vi "CheckCameraAttributes-CDH.vi"(2 "error in":errorcluster, 3 "Camera Name":T1) -> (0 "error out":errorcluster, 1 "Session Out":T1)   [LabVIEW 2013]
doc: "The Grab and Attributes Setup VI acquires images continuously and displays the images in an image control using high-level acquisition VIs. The VI also modifes the camera attributes while acquiring images. A grab is appropriate for high-speed applications in which you need to process only one image at a time."
uses:
  <vilib>/userdefined/High Color/IMAQdx.ctl
  <vilib>/vision/driver/IMAQdx.llb/IMAQdx Attribute Type.ctl
  <vilib>/vision/driver/IMAQdx.llb/IMAQdx Attribute Visibility.ctl
  <vilib>/vision/driver/NI_Vision_Acquisition_Software.lvlib
  <resource>/objmgr/imaqdx.rc
panel:
  out "Trigger::TriggerSource":string
  out "Trigger::TriggerParameter":dbl
  out "TriggerDelay::Value":dbl
  out "Trigger::TriggerActivation":string
  out "Shutter::Value":dbl
  out "Sharpness::Value":dbl
  out "Gamma::Value":dbl
  out "Gain::Value":dbl
  out "FrameRate::Value":dbl
  out "Brightness::Value":dbl
  out "AutoExposure::Value":dbl
  out "TriggerDelay::Mode":string
  out "Trigger::TriggerMode":string
  out "Shutter::Mode":string
  out "Sharpness::Mode":string
  out "Gamma::Mode":string
  out "Gain::Mode":string
  out "FrameRate::Mode":string
  out "Brightness::Mode":string
  out "AutoExposure::Mode":string
  out "PayloadSize":u32
  out "OverwriteMode":u32(ring) items=["Get Oldest"=0, "Fail"=2, "Get Newest"=3]
  out "ShiftPixelBits":bool
  out "Packet Size":u32
  out "Speed":u32
  out "SwapPixelBytes":bool
  out "PixelSignedness":u32
  out "Timeout":u32
  out "PixelFormat":u32
  out "BitsPerPixel":u32
  out "OffsetY":u32
  out "OffsetX":u32
  out "Width":u32
  out "Height":u32
  out "VideoMode":u32
  out "Current Mode":u32
  out "Video Modes":T2(array[cluster])
  in  "stop":bool
  in  "Get Button":bool
  out "Error While":errorcluster
  out "Attribute Information Array":T4(array[cluster])
  # "While the values at left are \"Enum\" type, the Property Node only accepts U32 values. \nTo figure out correspondence between number and setting, I had to setup the camera in NIMAX, save the settings (making them defualt) and then use my \"Get Camera Attributes.\""
  # "Ignore \"value\" if Mode=\"off\"!"
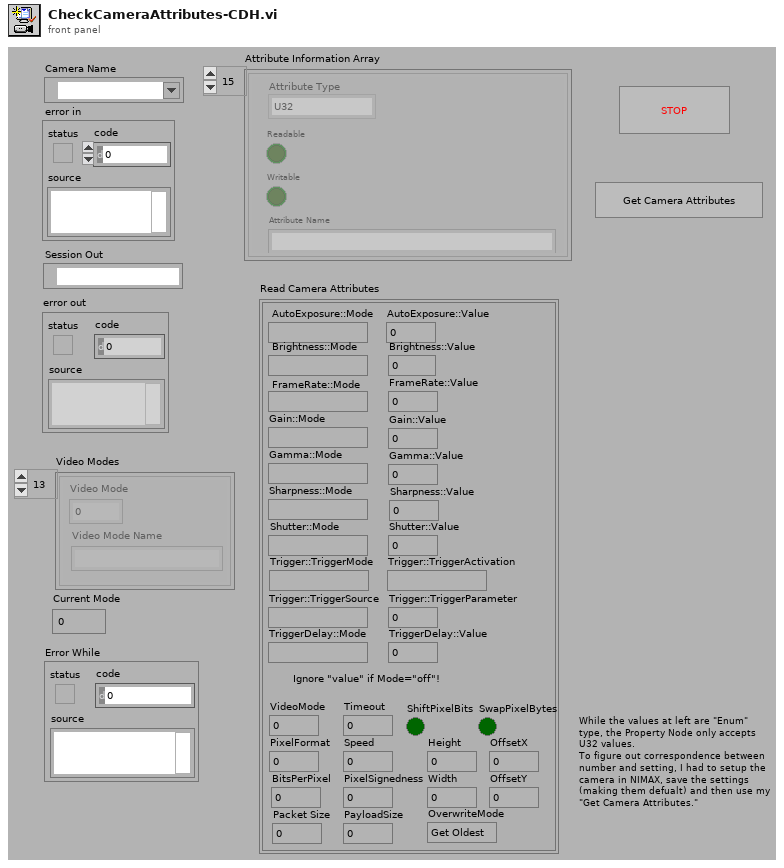
[diagram p1: front panel]
types:
  T1 = typedef "IMAQdx.ctl" = refnum<k21>
  T2 = cluster{"Video Mode":u32, "Video Mode Name":string}[]
  T3 = typedef "NI_Vision_Acquisition_Software.lvlib/IMAQdx Attribute Type.ctl" = enum32{"U32", "I64", "DBL", "String", "Enum", "Bool", "Command"}
  T4 = cluster{"Attribute Type":T3, "Readable":bool, "Writable":bool, "Attribute Name":string}[]
  T5 = typedef "NI_Vision_Acquisition_Software.lvlib/IMAQdx Attribute Visibility.ctl" = enum32{"Simple", "Intermediate", "Advanced"}
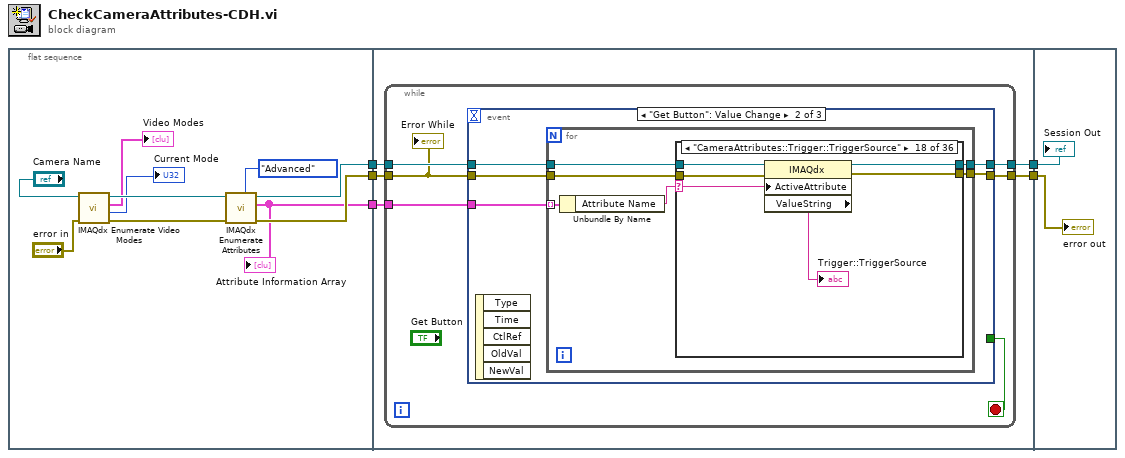
[diagram p0: block diagram]
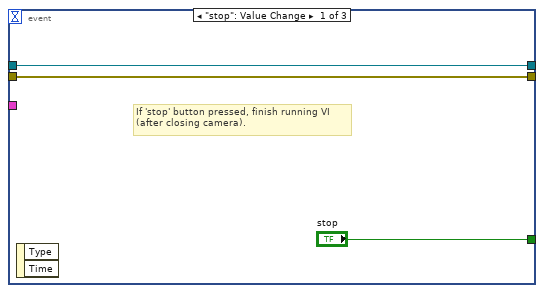
[diagram p2: hidden frame]
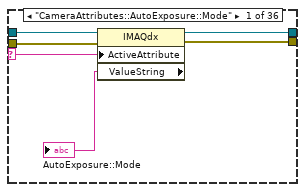
[diagram p3: hidden frame]
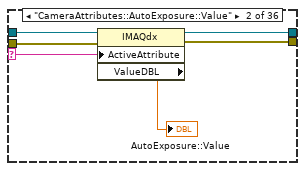
[diagram p4: hidden frame]
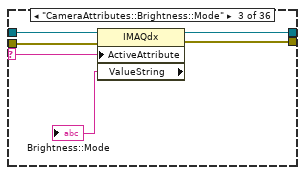
[diagram p5: hidden frame]
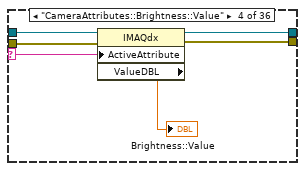
[diagram p6: hidden frame]
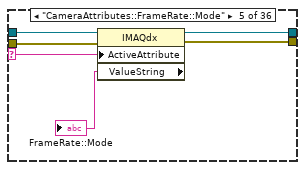
[diagram p7: hidden frame]
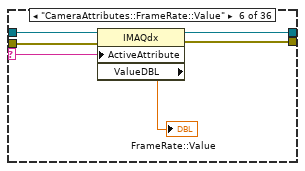
[diagram p8: hidden frame]
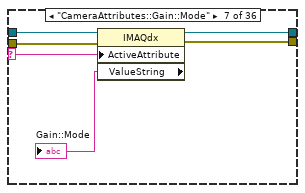
[diagram p9: hidden frame]
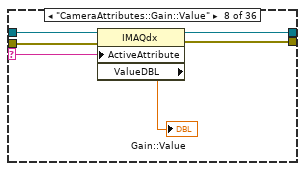
[diagram p10: hidden frame]
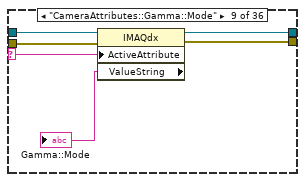
[diagram p11: hidden frame]
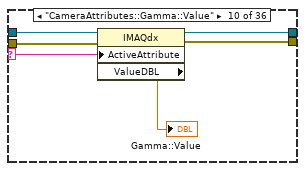
[diagram p12: hidden frame]
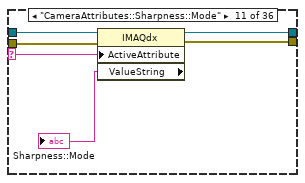
[diagram p13: hidden frame]
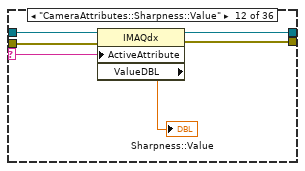
[diagram p14: hidden frame]
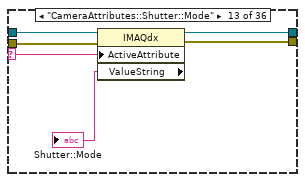
[diagram p15: hidden frame]
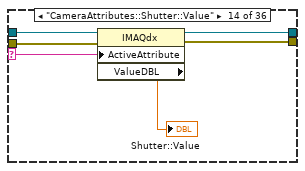
[diagram p16: hidden frame]
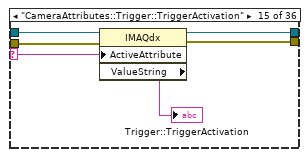
[diagram p17: hidden frame]
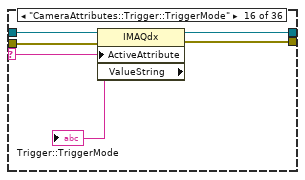
[diagram p18: hidden frame]
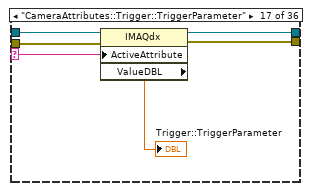
[diagram p19: hidden frame]
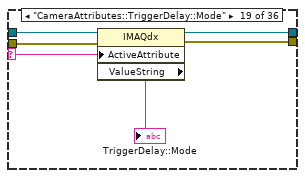
[diagram p20: hidden frame]
diagram:
  n1 = flat-sequence {
    tunnel: [w14] -> w5
    tunnel: [w10] -> w4
    tunnel: [w13] -> w1
    tunnel: w5 -> [w20]
    tunnel: w4 -> [w19]
    tunnel: [w18] -> w3
    tunnel: [w17] -> w2
    tunnel: w1 -> [w16]
    tunnel: w3 -> [w241]
    tunnel: w2 -> [w240]
    frame #0 {
      n2 = call <vilib>:"IMAQdx Enumerate Video Modes.vi"("error in"="error in", "Session In"="Camera Name") -> ("error out"=w11:errorcluster, "Current Mode"=→"Current Mode":u32, "Video Modes"=→"Video Modes":T2, "Session Out"=w12:T1)  [unwired: 6 in]
      n3 = call <vilib>:"IMAQdx Enumerate Attributes.vi"("Visibility"=IMAQdx_Attribute_Visibility."Advanced", "error in"=w11, "Session In"=w12) -> ("error out"=w14:errorcluster, "Attribute Information Array"=w13:T4, "Session Out"=w10:T1)  [unwired: 1 in, 5 out]
      "Attribute Information Array" <- w13
    }
    frame #1 {
      n4 = while {
        tunnel: w19 -> [w26]
        tunnel: [w25] -> w18
        tunnel: w20 -> [w24]
        tunnel: [w23] -> w17
        tunnel: w16 -> [w21]
        stop <- w22 stop-if-true
        n5 = event shown="[1] \"Get Button\": Value Change" {
          selector: _ -> [_ _ _]
          dyn-events: _ -> [_ _ _]
          timeout: _ -> [_ _ _]
          tunnel: [w28 w31 w239] -> w25
          tunnel: w26 -> [w28 w34 w239]
          tunnel: w24 -> [w27 w33 w238]
          tunnel: [w27 w30 w238] -> w23
          tunnel: ["stop" _ _] -> w22
          tunnel: w21 -> [_ w32 _]
          event "stop": Value Change {
            # "If 'stop' button pressed, finish running VI\n(after closing camera)."
            n6 = event-data() -> ()  [unwired: 1 in, 2 out]
          }
          event "Get Button": Value Change {
            n7 = event-data() -> ()  [unwired: 1 in, 5 out]
            n8 = for {
              tunnel: w34 -> [w38]
              tunnel: w33 -> [w37]
              tunnel: w32 -> [w40] mode=indexing
              tunnel: [w36] -> w31
              tunnel: [w35] -> w30
              n9 = Unbundle By Name(w40) -> ("Attribute Name"=w39:string)
              n10 = case shown="\"CameraAttributes::Trigger::TriggerSource\"" w39 {
                selector: w39 -> [w42 w48 w54 w60 w66 w72 w78 w84 w90 w96 w102 w108 w114 w120 w126 w132 w138 w144 w150 w156 _ _ _ _ _ _ _ _ _ _ _ _ _ _ _ _]
                tunnel: w38 -> [w46 w52 w58 w64 w70 w76 w82 w88 w94 w100 w106 w112 w118 w124 w130 w136 w142 w148 w154 w160 w165 w170 w175 w180 w185 w190 w195 w200 w205 w210 w215 w220 w225 w230 w235 w237]
                tunnel: w37 -> [w45 w51 w57 w63 w69 w75 w81 w87 w93 w99 w105 w111 w117 w123 w129 w135 w141 w147 w153 w159 w164 w169 w174 w179 w184 w189 w194 w199 w204 w209 w214 w219 w224 w229 w234 w236]
                tunnel: [w44 w50 w56 w62 w68 w74 w80 w86 w92 w98 w104 w110 w116 w122 w128 w134 w140 w146 w152 w158 w163 w168 w173 w178 w183 w188 w193 w198 w203 w208 w213 w218 w223 w228 w233 w237] -> w36
                tunnel: [w43 w49 w55 w61 w67 w73 w79 w85 w91 w97 w103 w109 w115 w121 w127 w133 w139 w145 w151 w157 w162 w167 w172 w177 w182 w187 w192 w197 w202 w207 w212 w217 w222 w227 w232 w236] -> w35
                frame "CameraAttributes::AutoExposure::Mode" {
                  n11 = property class="IMAQdx"(reference=w46, error in=w45, "ActiveAttribute"=w42) -> (reference out=w44:T1, error out=w43:errorcluster, "ValueString"=→"AutoExposure::Mode":string)
                }
                frame "CameraAttributes::AutoExposure::Value" {
                  n12 = property class="IMAQdx"(reference=w52, error in=w51, "ActiveAttribute"=w48) -> (reference out=w50:T1, error out=w49:errorcluster, "ValueDBL"=→"AutoExposure::Value":dbl)
                }
                frame "CameraAttributes::Brightness::Mode" {
                  n13 = property class="IMAQdx"(reference=w58, error in=w57, "ActiveAttribute"=w54) -> (reference out=w56:T1, error out=w55:errorcluster, "ValueString"=→"Brightness::Mode":string)
                }
                frame "CameraAttributes::Brightness::Value" {
                  n14 = property class="IMAQdx"(reference=w64, error in=w63, "ActiveAttribute"=w60) -> (reference out=w62:T1, error out=w61:errorcluster, "ValueDBL"=→"Brightness::Value":dbl)
                }
                frame "CameraAttributes::FrameRate::Mode" {
                  n15 = property class="IMAQdx"(reference=w70, error in=w69, "ActiveAttribute"=w66) -> (reference out=w68:T1, error out=w67:errorcluster, "ValueString"=→"FrameRate::Mode":string)
                }
                frame "CameraAttributes::FrameRate::Value" {
                  n16 = property class="IMAQdx"(reference=w76, error in=w75, "ActiveAttribute"=w72) -> (reference out=w74:T1, error out=w73:errorcluster, "ValueDBL"=→"FrameRate::Value":dbl)
                }
                frame "CameraAttributes::Gain::Mode" {
                  n17 = property class="IMAQdx"(reference=w82, error in=w81, "ActiveAttribute"=w78) -> (reference out=w80:T1, error out=w79:errorcluster, "ValueString"=→"Gain::Mode":string)
                }
                frame "CameraAttributes::Gain::Value" {
                  n18 = property class="IMAQdx"(reference=w88, error in=w87, "ActiveAttribute"=w84) -> (reference out=w86:T1, error out=w85:errorcluster, "ValueDBL"=→"Gain::Value":dbl)
                }
                frame "CameraAttributes::Gamma::Mode" {
                  n19 = property class="IMAQdx"(reference=w94, error in=w93, "ActiveAttribute"=w90) -> (reference out=w92:T1, error out=w91:errorcluster, "ValueString"=→"Gamma::Mode":string)
                }
                frame "CameraAttributes::Gamma::Value" {
                  n20 = property class="IMAQdx"(reference=w100, error in=w99, "ActiveAttribute"=w96) -> (reference out=w98:T1, error out=w97:errorcluster, "ValueDBL"=→"Gamma::Value":dbl)
                }
                frame "CameraAttributes::Sharpness::Mode" {
                  n21 = property class="IMAQdx"(reference=w106, error in=w105, "ActiveAttribute"=w102) -> (reference out=w104:T1, error out=w103:errorcluster, "ValueString"=→"Sharpness::Mode":string)
                }
                frame "CameraAttributes::Sharpness::Value" {
                  n22 = property class="IMAQdx"(reference=w112, error in=w111, "ActiveAttribute"=w108) -> (reference out=w110:T1, error out=w109:errorcluster, "ValueDBL"=→"Sharpness::Value":dbl)
                }
                frame "CameraAttributes::Shutter::Mode" {
                  n23 = property class="IMAQdx"(reference=w118, error in=w117, "ActiveAttribute"=w114) -> (reference out=w116:T1, error out=w115:errorcluster, "ValueString"=→"Shutter::Mode":string)
                }
                frame "CameraAttributes::Shutter::Value" {
                  n24 = property class="IMAQdx"(reference=w124, error in=w123, "ActiveAttribute"=w120) -> (reference out=w122:T1, error out=w121:errorcluster, "ValueDBL"=→"Shutter::Value":dbl)
                }
                frame "CameraAttributes::Trigger::TriggerActivation" {
                  n25 = property class="IMAQdx"(reference=w130, error in=w129, "ActiveAttribute"=w126) -> (reference out=w128:T1, error out=w127:errorcluster, "ValueString"=→"Trigger::TriggerActivation":string)
                }
                frame "CameraAttributes::Trigger::TriggerMode" {
                  n26 = property class="IMAQdx"(reference=w136, error in=w135, "ActiveAttribute"=w132) -> (reference out=w134:T1, error out=w133:errorcluster, "ValueString"=→"Trigger::TriggerMode":string)
                }
                frame "CameraAttributes::Trigger::TriggerParameter" {
                  n27 = property class="IMAQdx"(reference=w142, error in=w141, "ActiveAttribute"=w138) -> (reference out=w140:T1, error out=w139:errorcluster, "ValueDBL"=→"Trigger::TriggerParameter":dbl)
                }
                frame "CameraAttributes::Trigger::TriggerSource" {
                  n28 = property class="IMAQdx"(reference=w148, error in=w147, "ActiveAttribute"=w144) -> (reference out=w146:T1, error out=w145:errorcluster, "ValueString"=→"Trigger::TriggerSource":string)
                }
                frame "CameraAttributes::TriggerDelay::Mode" {
                  n29 = property class="IMAQdx"(reference=w154, error in=w153, "ActiveAttribute"=w150) -> (reference out=w152:T1, error out=w151:errorcluster, "ValueString"=→"TriggerDelay::Mode":string)
                }
                frame "CameraAttributes::TriggerDelay::Value" {
                  n30 = property class="IMAQdx"(reference=w160, error in=w159, "ActiveAttribute"=w156) -> (reference out=w158:T1, error out=w157:errorcluster, "ValueDBL"=→"TriggerDelay::Value":dbl)
                }
                frame "AcquisitionAttributes::VideoMode" {
                  n31 = property class="IMAQdx"(reference=w165, error in=w164) -> (reference out=w163:T1, error out=w162:errorcluster, "VideoMode"=→"VideoMode":u32)
                }
                frame "AcquisitionAttributes::BitsPerPixel" {
                  n32 = property class="IMAQdx"(reference=w170, error in=w169) -> (reference out=w168:T1, error out=w167:errorcluster, "BitsPerPixel"=→"BitsPerPixel":u32)
                }
                frame "AcquisitionAttributes::PixelFormat" {
                  n33 = property class="IMAQdx"(reference=w175, error in=w174) -> (reference out=w173:T1, error out=w172:errorcluster, "PixelFormat"=→"PixelFormat":u32)
                }
                frame "AcquisitionAttributes::Timeout" {
                  n34 = property class="IMAQdx"(reference=w180, error in=w179) -> (reference out=w178:T1, error out=w177:errorcluster, "Timeout"=→"Timeout":u32)
                }
                frame "AcquisitionAttributes::PixelSignedness" {
                  n35 = property class="IMAQdx"(reference=w185, error in=w184) -> (reference out=w183:T1, error out=w182:errorcluster, "PixelSignedness"=→"PixelSignedness":u32)
                }
                frame "AcquisitionAttributes::Speed" {
                  n36 = property class="IMAQdx"(reference=w190, error in=w189) -> (reference out=w188:T1, error out=w187:errorcluster, "Speed"=→"Speed":u32)
                }
                frame "AcquisitionAttributes::SwapPizelBytes" {
                  n37 = property class="IMAQdx"(reference=w195, error in=w194) -> (reference out=w193:T1, error out=w192:errorcluster, "SwapPixelBytes"=→"SwapPixelBytes":bool)
                }
                frame "AcquisitionAttributes::Height" {
                  n38 = property class="IMAQdx"(reference=w200, error in=w199) -> (reference out=w198:T1, error out=w197:errorcluster, "Height"=→"Height":u32)
                }
                frame "AcquisitionAttributes::Width" {
                  n39 = property class="IMAQdx"(reference=w205, error in=w204) -> (reference out=w203:T1, error out=w202:errorcluster, "Width"=→"Width":u32)
                }
                frame "AcquisitionAttributes::OffsetX" {
                  n40 = property class="IMAQdx"(reference=w210, error in=w209) -> (reference out=w208:T1, error out=w207:errorcluster, "OffsetX"=→"OffsetX":u32)
                }
                frame "AcquisitionAttributes::OffsetY" {
                  n41 = property class="IMAQdx"(reference=w215, error in=w214) -> (reference out=w213:T1, error out=w212:errorcluster, "OffsetY"=→"OffsetY":u32)
                }
                frame "AcquisitionAttributes::PacketSize" {
                  n42 = property class="IMAQdx"(reference=w220, error in=w219) -> (reference out=w218:T1, error out=w217:errorcluster, "PacketSize"=→"Packet Size":u32)
                }
                frame "AcquisitionAttributes::PayloadSize" {
                  n43 = property class="IMAQdx"(reference=w225, error in=w224) -> (reference out=w223:T1, error out=w222:errorcluster, "PayloadSize"=→"PayloadSize":u32)
                }
                frame "AcquisitionAttributes::ShiftPixelBits" {
                  n44 = property class="IMAQdx"(reference=w230, error in=w229) -> (reference out=w228:T1, error out=w227:errorcluster, "ShiftPixelBits"=→"ShiftPixelBits":bool)
                }
                frame "AcquisitionAttributes::OverwriteMode" {
                  n45 = property class="IMAQdx"(reference=w235, error in=w234) -> (reference out=w233:T1, error out=w232:errorcluster, "OverwriteMode"=→"OverwriteMode":u32)
                }
                frame Default {
                }
              }
            }
          }
          event Timeout {
            n46 = event-data() -> ()  [unwired: 1 in, 2 out]
          }
        }
        "Error While" <- w24
      }
    }
    frame #2 {
      "error out" <- w240
      "Session Out" <- w241
    }
  }
